vi "LibXML_Validate.vi"(8 "error in":errorcluster, 9 "validate against URI":string, 10 "validation type":enum16{"DTD", "Schema", "RelaxNG"}(ring), 11 "doc in":u32) -> (0 "error out":errorcluster, 1 "valid!":bool, 3 "doc out":u32)   [LabVIEW 2019, in "Tools.lvlib" / "LibXML.lvlib"]
doc: "Validates XML against URI"
uses:
  LibXML.lvlib
  dll/lXMLwrap.dll
panel:
  out "output param":i32
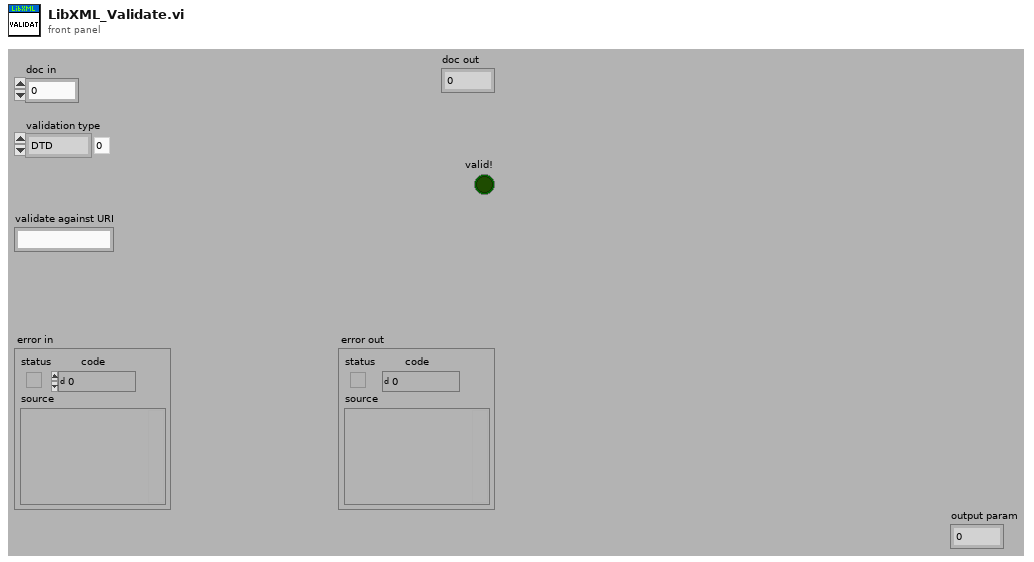
[diagram p1: front panel]
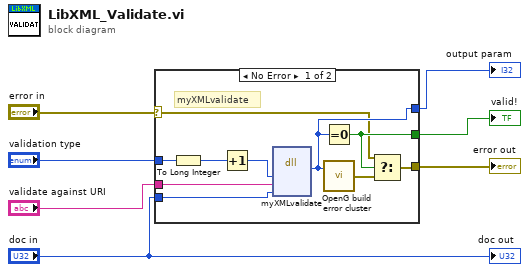
[diagram p0: block diagram]
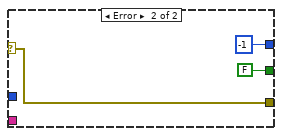
[diagram p2: hidden frame]
diagram:
  n1 = case shown="No Error" "error in" {
    selector: "error in" -> [w8 w20]
    tunnel: [w16 w20] -> w7
    tunnel: [w14 FALSE ("parsed")] -> w6
    tunnel: "doc in" -> [w15 _]
    tunnel: [w12 -1 ("return type")] -> w3
    tunnel: "validation type" -> [w11 _]
    tunnel: "validate against URI" -> [w10 _]
    frame No Error {
      # "myXMLvalidate"
      n2 = To Long Integer(number=w11) -> (32bit integer=w9:i32)
      n3 = Increment(x=w9) -> (x+1=w13:i32)
      n4 = dll-call lib="C:/Projects/_Prywatne/MyCIT/Framework/Tools/XML/LibXML/dll/lXMLwrap.dll" fn="myXMLvalidate"("type"=w13, "againstFile"=w10, "doc"=w15) -> ("return type"=w12:i32)  [unwired: 6 in, 2 out]
      n5 = Equal To 0?(x=w12) -> (x = 0?=w14:bool)
      n6 = call "OpenG build error cluster.vi"("code"=w12) -> ("error out"=w17:errorcluster)  [unwired: 1 in]
      n7 = Select(t=w8, s=w14, f=w17) -> (s? t:f=w16:errorcluster)
    }
    frame Error {
    }
  }
  "error out" <- w7
  "valid!" <- w6
  "output param" <- w3
  "doc out" <- "doc in"
